vi "Error Log.vi"(8 "error in":errorcluster, 10 "Level":string, 11 "error happened":errorcluster) -> (0 "error out":errorcluster)   [LabVIEW 2020]
panel:
  # "Not sure what level means so we will clarify later"
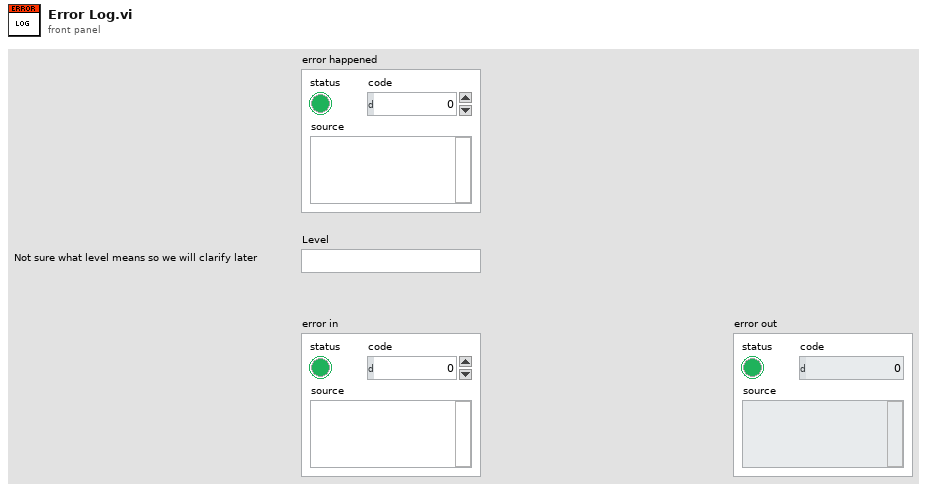
[diagram p1: front panel]
types:
  T1 = enum16{"open", "replace", "create", "open or create", "replace or create", "replace or create with confirmation"}
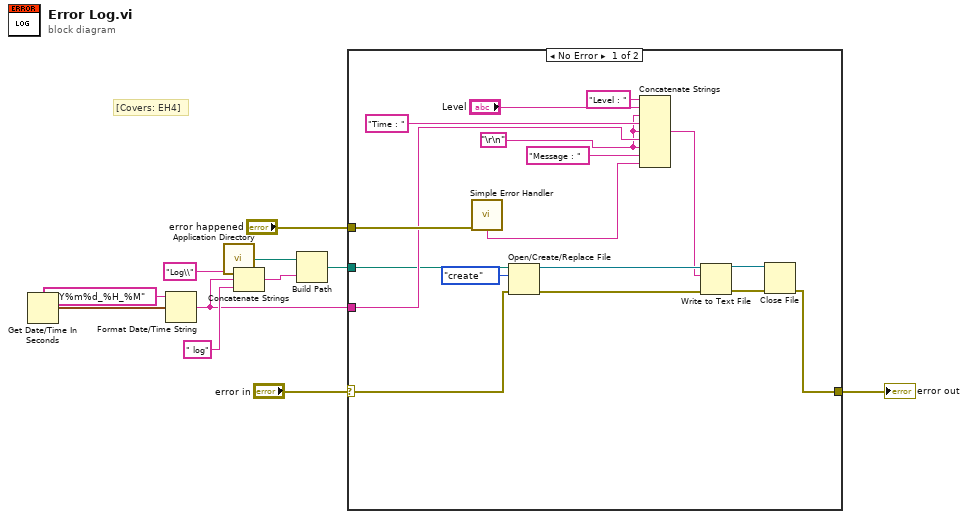
[diagram p0: block diagram]
diagram:
  # "[Covers: EH4]"
  n1 = Get Date/Time In Seconds() -> (seconds since 1Jan1904=w5:timestamp)
  n2 = Format Date/Time String(time format string (%c)="%Y%m%d_%H_%M", seconds (now)=w5) -> (date/time string=w1:string)  [unwired: 1 in]
  n3 = call <vilib>:"Application Directory.vi"() -> ("Application Directory"=w8:path)
  n4 = Concatenate Strings("Log\\" ("string"), w1, " log" ("string")) -> (w6:string)
  n5 = Build Path(base path=w8, name or relative path=w6) -> (appended path=w3:path)
  n6 = case shown="No Error" "error in" {
    selector: "error in" -> [w13 w29]
    tunnel: [w12 w29] -> w10
    tunnel: "error happened" -> [w28 _]
    tunnel: w3 -> [w20 _]
    tunnel: w1 -> [w25 _]
    frame No Error {
      w23 = "\r\n"
      n7 = call <vilib>:"Simple Error Handler.vi"("error in (no error)"=w28) -> ("message"=w26:string)  [unwired: 4 in, 4 out]
      n8 = Open/Create/Replace File(file path (use dialog)=w20, error in=w13, operation (0:open)=T1."create") -> (refnum out=w19:refnum<file>, error out=w18:errorcluster)  [unwired: 3 in, 1 out]
      n9 = Concatenate Strings("Level : " ("string"), "Level", w23, "Time : " ("string"), w23, w25, w23, "Message : " ("string"), w26) -> (w17:string)
      n10 = Write to Text File(file (use dialog)=w19, text=w17, error in=w18) -> (refnum out=w15:refnum<file>, error out=w14:errorcluster)  [unwired: 1 in, 1 out]
      n11 = Close File(refnum=w15, error in=w14) -> (error out=w12:errorcluster)  [unwired: 1 out]
    }
    frame Error {
    }
  }
  "error out" <- w10
